vi "Serialize Boolean.vi"(3 "data":bool) -> (1 "bytes":u8[](array[numeric]))   [LabVIEW 2020, in "NI_SFTP.lvlib" / "Low Level Connection.lvclass"]
uses:
  <vilib>/net/SFTP/Low Level Connection/Low Level Connection.lvclass
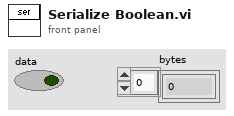
[diagram p1: front panel]
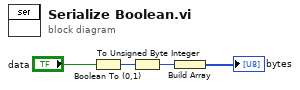
[diagram p0: block diagram]
diagram:
  n1 = Boolean To (0,1)(Boolean="data") -> (0, 1=w2:i16)
  n2 = To Unsigned Byte Integer(number=w2) -> (unsigned 8bit integer=w1:u8)
  n3 = Build Array(w1) -> (→"bytes":u8[])
